vi "Write Umgebung.Zustandsgrössen.vi"(8 "error in (no error)":errorcluster, 10 "Umgebung.Zustandsgrössen":T1, 11 "Umgebung in":refnum<class "Umgebung.lvclass">) -> (0 "error out":errorcluster, 3 "Umgebung out":refnum<class "Umgebung.lvclass">)   [LabVIEW 2016, in "Umgebung.lvclass"]
uses:
  Umgebung.lvclass
  Umgebung.lvclass/Umgebung.ctl
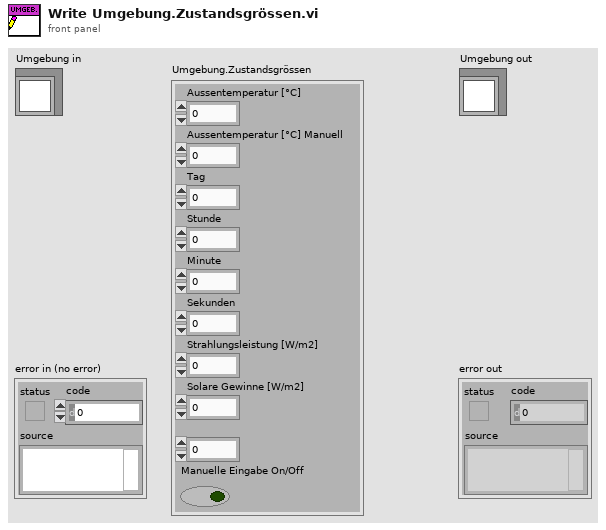
[diagram p1: front panel]
types:
  T1 = typedef "Umgebung.lvclass/Umgebung.Zustandsgrössen.ctl" = cluster{"Aussentemperatur [°C]":dbl, "Aussentemperatur [°C] Manuell":dbl, "Tag":dbl, "Stunde":dbl, "Minute":dbl, "Sekunden":dbl, "Strahlungsleistung [W/m2]":dbl, "Solare Gewinne [W/m2]":dbl, "Solare Gewinne [W/m2] Manuell":dbl, "Manuelle Eingabe On/Off":bool}
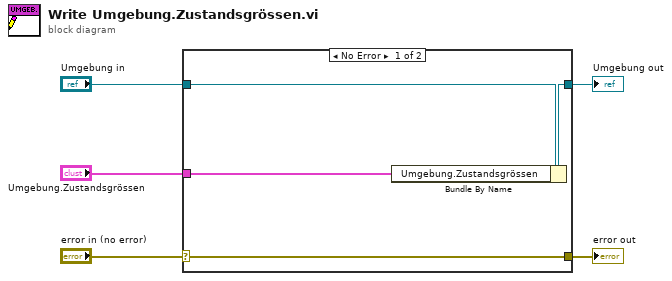
[diagram p0: block diagram]
diagram:
  n1 = case shown="No Error" "error in (no error)" {
    selector: "error in (no error)" -> [w9 w10]
    tunnel: [w9 w10] -> w4
    tunnel: [w7 w11] -> w2
    tunnel: "Umgebung in" -> [w8 w11]
    tunnel: "Umgebung.Zustandsgrössen" -> [w6 _]
    frame No Error {
      n2 = Bundle By Name(cluster=w8, "Umgebung.Zustandsgrössen"=w6) -> (w7:refnum<class "Umgebung.lvclass">)
    }
    frame Error {
    }
  }
  "error out" <- w4
  "Umgebung out" <- w2
